vi "Image Acquisition Settings from ini.vi"(7 "Section":string, 8 "error in (no error)":errorcluster, 11 "Acquisition Settings In":T1={"Image Width"=2040, "Image Height"=1088, "Frames To Acquire"=0, "Signal Mapping"=enum."Basler 10-tap", "DMA Buffer Size\n(In Images)"=64} {"Image Height" max=65535; "Image Width" max=65535 step=40}) -> (0 "error out":errorcluster, 3 "Acquisition Settings Cluster":T1={"Image Width"=2040, "Image Height"=1088, "Frames To Acquire"=0, "Signal Mapping"=enum."Basler 10-tap", "DMA Buffer Size\n(In Images)"=64} {"Image Height" max=65535; "Image Width" max=65535 step=40}, 5 "All Tags Exists?":bool)   [LabVIEW 2013]
doc: "Loads the TCP port being used for listening for incoming connections."
uses:
  Image Acquisition/Acquisition Settings Cluster.ctl
  Image Acquisition Setting Enum Keys.ctl
  Common/File IO/INI/Read write mode.ctl
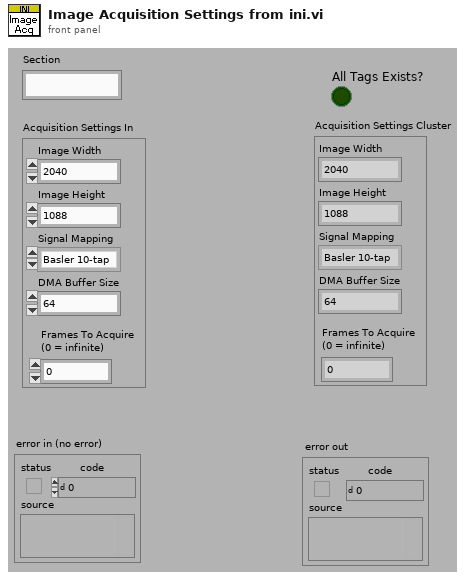
[diagram p1: front panel]
types:
  T1 = typedef "Acquisition Settings Cluster.ctl" = cluster{"Image Width":u32, "Image Height":u32, "Frames To Acquire":u32, "Signal Mapping":enum8{"Standard", "Basler 10-tap", "Vosskühler 10-tap"}, "DMA Buffer Size\n(In Images)":u32}
  T2 = typedef "Image Acquisition Setting Enum Keys.ctl" = enum16{"Height", "Width", "DMA Buffer Size"}
  T3 = typedef "Read write mode.ctl" = enum16{"Read", "Write"}
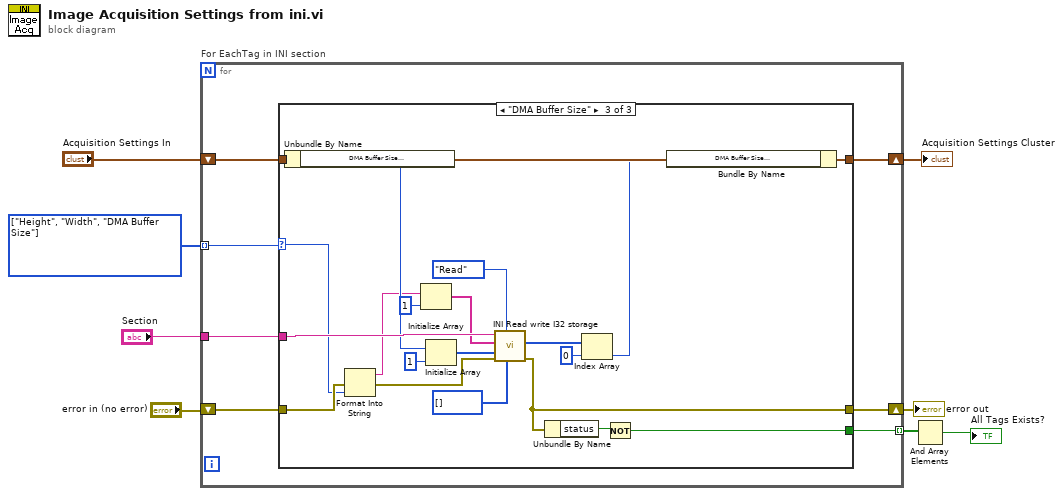
[diagram p0: block diagram]
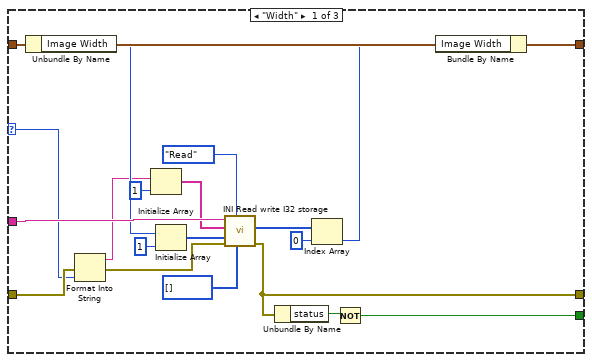
[diagram p2: hidden frame]
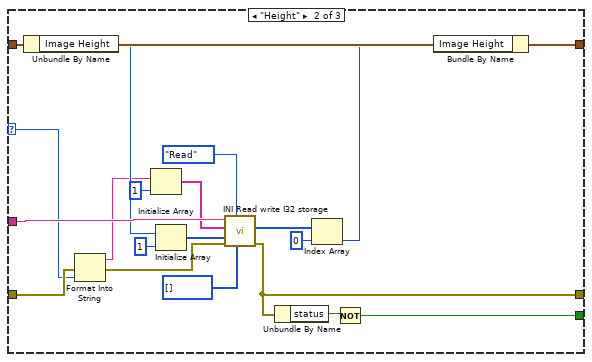
[diagram p3: hidden frame]
diagram:
  w8 = T2[] [enum."Height", enum."Width", enum."DMA Buffer Size"] items=["Height", "Width", "DMA Buffer Size"]
  n1 = for "For EachTag in INI section" {
    tunnel: "Section" -> [w15]
    tunnel: w8 -> [w14] mode=indexing
    shift-right: [w10] -> w6
    shift-left: "error in (no error)" -> [w12]
    shift-right: [w9] -> w1
    shift-left: "Acquisition Settings In" -> [w13]
    tunnel: [w11] -> w4 mode=indexing
    n2 = case shown="\"DMA Buffer Size\"" w14 {
      selector: w14 -> [w30 w50 w70]
      tunnel: w15 -> [w34 w54 w74]
      tunnel: w13 -> [w32 w52 w72]
      tunnel: w12 -> [w31 w51 w71]
      tunnel: [w35 w55 w75] -> w10
      tunnel: [w17 w37 w57] -> w11
      tunnel: [w33 w53 w73] -> w9
      frame "Width" {
        n3 = Unbundle By Name(w32) -> ("Image Width"=w28:u32)
        n4 = Format Into String(error in=w31, w30) -> (resulting string=w25:string, error out=w18:errorcluster)  [unwired: 2 in]
        n5 = Initialize Array(w25, 1 ("dimension size")) -> (w23:string[])
        n6 = Initialize Array(w28, 1 ("dimension size")) -> (w26:u32[])
        n7 = call "INI Read write I32 storage.vi"("Values to write"=i32[] [], "Read/Write mode"=Read_write_mode."Read", "error in"=w18, "Defaults"=w26, "keys"=w23, "section"=w34) -> ("error out"=w35:errorcluster, "Values"=w22:i32[])  [unwired: 4 in]
        n8 = Unbundle By Name(w35) -> ("status"=w19:bool)
        n9 = Index Array(array=w22, index=0) -> (element=w20:i32)
        n10 = Not(x=w19) -> (.not. x?=w17:bool)
        n11 = Bundle By Name(cluster=w32, "Image Width"=w20) -> (w33:T1)
      }
      frame "Height" {
        n12 = Unbundle By Name(w52) -> ("Image Height"=w48:u32)
        n13 = Format Into String(error in=w51, w50) -> (resulting string=w45:string, error out=w38:errorcluster)  [unwired: 2 in]
        n14 = Initialize Array(w45, 1 ("dimension size")) -> (w43:string[])
        n15 = Initialize Array(w48, 1 ("dimension size")) -> (w46:u32[])
        n16 = call "INI Read write I32 storage.vi"("Values to write"=i32[] [], "Read/Write mode"=Read_write_mode."Read", "error in"=w38, "Defaults"=w46, "keys"=w43, "section"=w54) -> ("error out"=w55:errorcluster, "Values"=w42:i32[])  [unwired: 4 in]
        n17 = Unbundle By Name(w55) -> ("status"=w39:bool)
        n18 = Index Array(array=w42, index=0) -> (element=w40:i32)
        n19 = Not(x=w39) -> (.not. x?=w37:bool)
        n20 = Bundle By Name(cluster=w52, "Image Height"=w40) -> (w53:T1)
      }
      frame "DMA Buffer Size" {
        n21 = Unbundle By Name(w72) -> ("DMA Buffer Size\n(In Images)"=w68:u32)
        n22 = Format Into String(error in=w71, w70) -> (resulting string=w65:string, error out=w58:errorcluster)  [unwired: 2 in]
        n23 = Initialize Array(w65, 1 ("dimension size")) -> (w63:string[])
        n24 = Initialize Array(w68, 1 ("dimension size")) -> (w66:u32[])
        n25 = call "INI Read write I32 storage.vi"("Values to write"=i32[] [], "Read/Write mode"=Read_write_mode."Read", "error in"=w58, "Defaults"=w66, "keys"=w63, "section"=w74) -> ("error out"=w75:errorcluster, "Values"=w62:i32[])  [unwired: 4 in]
        n26 = Unbundle By Name(w75) -> ("status"=w59:bool)
        n27 = Index Array(array=w62, index=0) -> (element=w60:i32)
        n28 = Not(x=w59) -> (.not. x?=w57:bool)
        n29 = Bundle By Name(cluster=w72, "DMA Buffer Size\n(In Images)"=w60) -> (w73:T1)
      }
    }
  }
  "error out" <- w6
  "Acquisition Settings Cluster" <- w1
  n30 = And Array Elements(Boolean array=w4) -> (logical AND=→"All Tags Exists?":bool)
